vi "EmergencyConditions (1).vi"(8 "error in (no error)":errorcluster) -> (0 "error out":errorcluster)   [LabVIEW 2017]
doc: "Checks emergency conditions and if any are met, returns an error, prompting emergency protocol."
uses:
  Sensors/DataStreamIndex.ctl
  LoopPeriodGLOBAL.vi
  Emergency/EmergencyStringGLOBAL.vi
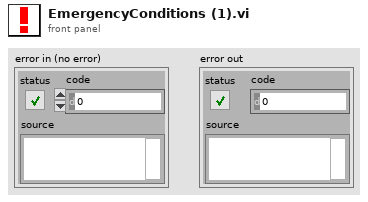
[diagram p1: front panel]
types:
  T1 = typedef "DataStreamIndex.ctl" = enum16{"SuspensionPT (PSI)", "MagBrakePT (PSI)", "Baby HPPT (PSI)", "BigRight HPPT (PSI)", "BigLeft HPPT (PSI)", "HallEffect FrontLeft (V)", "HallEffect FrontRight (V)", "HallEffect BackRight (V)", "HallEffect BackLeft (V)", "LinearPot FrontRight (V)", "LinearPot FrontLeft (V)", "LinearPot BackRight (V)", "LinearPot BackLeft (V)", "Speed (m/s)", "Distance (m)", "Piezo (V)", "Battery Voltage (V)", "Battery Current", "Battery Temperature (C)", "cRIO Temperature (C)", "Right Big Tank Temperature (C)", "Left Big Tank Temperature (C)", "Baby Tank Temperature (C)", "Right Manifold Temperature (C)", "Left Manifold Temperature (C)", "IMU Acceleration (m/s2)", "IMU Pressure (Pa)", "IMU Temperature (C)"}
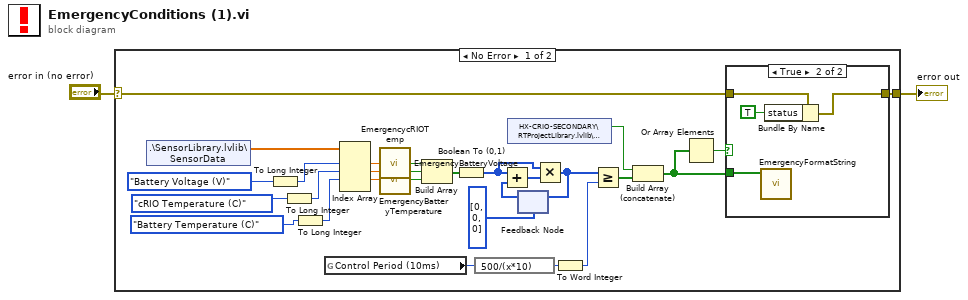
[diagram p0: block diagram]
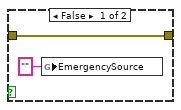
[diagram p2: hidden frame]
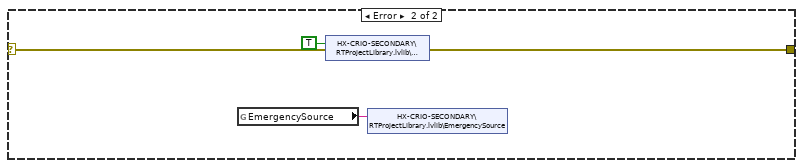
[diagram p3: hidden frame]
diagram:
  n1 = case shown="No Error" "error in (no error)" {
    selector: "error in (no error)" -> [w18 w39]
    tunnel: [w30 w39] -> w1
    frame No Error {
      n2 = shared-variable ".\\SensorLibrary.lvlib\\SensorData"() -> (w28:dbl[])  [unwired: 1 in, 1 out]
      n3 = To Long Integer(number=DataStreamIndex."Battery Voltage (V)" ("Data Stream Index")) -> (32bit integer=w27:i32)
      n4 = To Long Integer(number=DataStreamIndex."cRIO Temperature (C)" ("Data Stream Index")) -> (32bit integer=w26:i32)
      n5 = To Long Integer(number=DataStreamIndex."Battery Temperature (C)" ("Data Stream Index")) -> (32bit integer=w25:i32)
      n6 = global read "LoopPeriodGLOBAL.vi" "Control Period (10ms)"() -> (w12:i64)
      n7 = Index Array(array=w28, index #1=w27, index #2=w26, index #3=w25) -> (element #1=w24:dbl, element #2=w20:dbl, element #3=w22:dbl)  [unwired: 1 in, 1 out]
      n8 = call "EmergencyBatteryVoltage.vi"("Numeric"=w24) -> ("Boolean"=w23:bool)
      n9 = call "EmergencycRIOTemp.vi"("Numeric"=w20) -> ("Boolean"=w19:bool)
      n10 = call "EmergencyBatteryTemperature.vi"("Numeric"=w22) -> ("Boolean"=w21:bool)
      n11 = Build Array(w23, w19, w21) -> (w5:bool[])
      n12 = Boolean To (0,1)(Boolean=w5) -> (0, 1=w16:i16[])
      n13 = expression code="500/(x*10)"(w12) -> (w11:i64)
      n14 = shared-variable "HX-CRIO-SECONDARY\\RTProjectLibrary.lvlib\\Emergency"() -> (w8:bool)  [unwired: 1 in, 1 out]
      n15 = feedback #1(i16[] [0, 0, 0]) -> (w15:i16[])
      n16 = Add(x=w16, y=w15) -> (x+y=w17:i16[])
      n17 = Multiply(x=w16, y=w17) -> (x*y=w13:i16[])
      n18 = feedback-in #1(w13) -> ()
      n19 = To Word Integer(number=w11) -> (16bit integer=w10:i16)
      n20 = Greater Or Equal?(x=w13, y=w10) -> (x >= y?=w9:bool[])
      n21 = Build Array (concatenate)(w8, w9) -> (w6:bool[])
      n22 = Or Array Elements(Boolean array=w6) -> (logical OR=w7:bool)
      n23 = case shown="True" w7 {
        tunnel: w18 -> [w32 w36]
        tunnel: [w32 w35] -> w30
        tunnel: w6 -> [_ w33]
        frame False {
          n24 = global write "EmergencyStringGLOBAL.vi" "EmergencySource"("" ("EmergencySource")) -> ()
        }
        frame True {
          n25 = call "EmergencyFormatString.vi"("Array"=w33) -> ()  [unwired: 11 in]
          n26 = Bundle By Name(cluster=w36, "status"=TRUE) -> (w35:errorcluster)
        }
      }
    }
    frame Error {
      n27 = global read "EmergencyStringGLOBAL.vi" "EmergencySource"() -> (w37:string)
      n28 = shared-variable "HX-CRIO-SECONDARY\\RTProjectLibrary.lvlib\\Emergency"(TRUE ("Emergency")) -> ()  [unwired: 1 in, 1 out]
      n29 = shared-variable "HX-CRIO-SECONDARY\\RTProjectLibrary.lvlib\\EmergencySource"(w37) -> ()  [unwired: 1 in, 1 out]
    }
  }
  "error out" <- w1
